vi "TableToArrayFract32(SubVI).vi"(11 "String in":string) -> (2 "Array":fxp<+/-,32,1>[](array[numeric]))   [LabVIEW 2017, in "LV_Unicorn.lvlib"]
uses:
  LV_Unicorn.lvlib
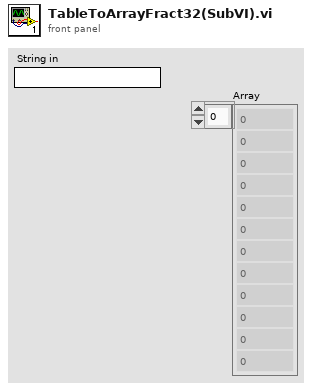
[diagram p1: front panel]
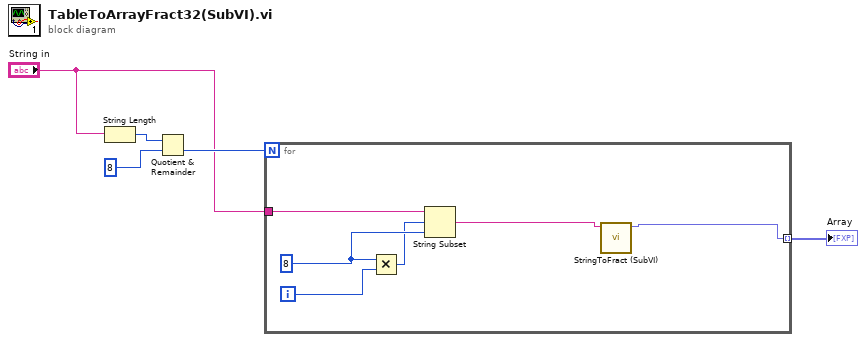
[diagram p0: block diagram]
diagram:
  n1 = String Length(string="String in") -> (length=w2:i32)
  n2 = Quotient & Remainder(x=w2, y=8) -> (floor(x/y)=w4:i32)  [unwired: 1 out]
  n3 = for {
    N: w4 -> [_]
    tunnel: "String in" -> [w11]
    tunnel: [w6] -> w5 mode=indexing
    i -> [w10]
    w9 = 8 ("length (rest)")
    n4 = Multiply(x=w9, y=w10) -> (x*y=w8:i32)
    n5 = String Subset(string=w11, offset (0)=w8, length (rest)=w9) -> (substring=w7:string)
    n6 = call "StringToFract (SubVI).vi"("String in"=w7) -> ("Numeric"=w6:fxp<+/-,32,1>)  [unwired: 10 in]
  }
  "Array" <- w5
